vi "DAQNavi Read (Counter 1D Pulse Width 1Chan NSamp).vi"(8 "error in (no error)":errorcluster, 9 "number of samples per channel to read":u32=10, 10 "timeout":dbl=10.0, 11 "task in":i32) -> (0 "error out":errorcluster, 2 "data":cluster{"high period":dbl, "low period":dbl}[](array[cluster]), 3 "task out":i32)   [LabVIEW 2020]
uses:
  DAQNavi_LV.dll
panel:
  in  "pulse width 2":cluster{"high period":dbl, "low period":dbl}
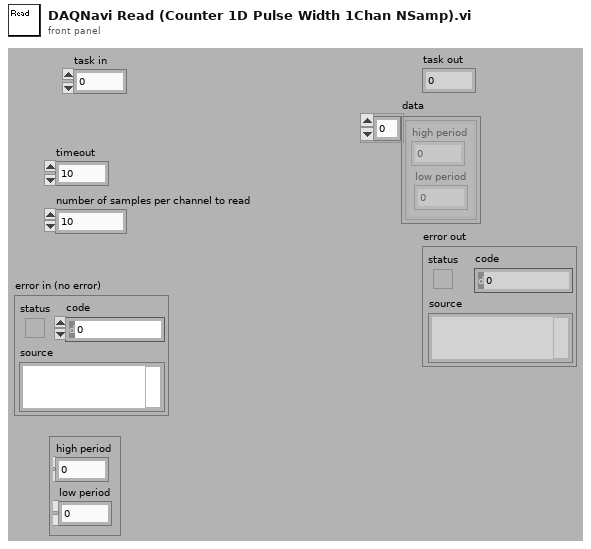
[diagram p1: front panel]
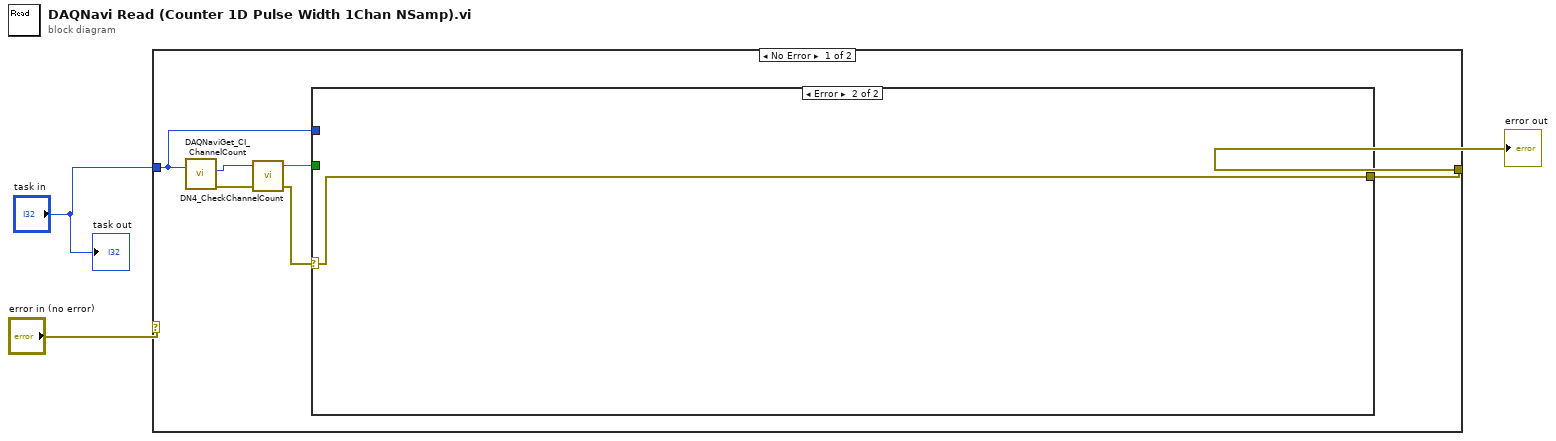
[diagram p0: block diagram]
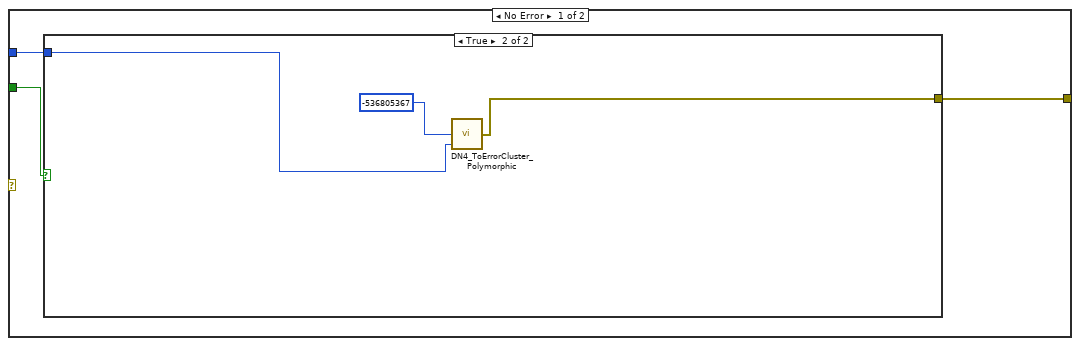
[diagram p2: hidden frame]
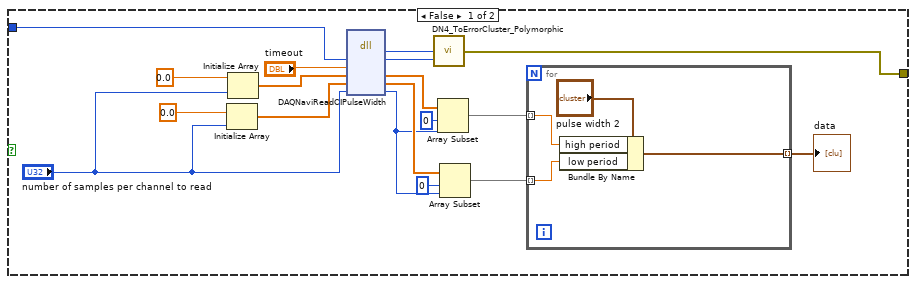
[diagram p3: hidden frame]
diagram:
  n1 = case shown="No Error" "error in (no error)" {
    selector: "error in (no error)" -> [_ w39]
    tunnel: [w9 w39] -> w2
    tunnel: "task in" -> [w4 _]
    frame No Error {
      n2 = call "DAQNaviGet_CI_ChannelCount.vi"("task in"=w4) -> ("error out"=w7:errorcluster, "channel count"=w8:i32)  [unwired: 1 in, 8 out]
      n3 = call "DN4_CheckChannelCount.vi"("error out"=w7, "channel count"=w8) -> ("error IO"=w6:errorcluster, "greater than 1?"=w5:bool)  [unwired: 2 out]
      n4 = case shown="Error" w6 {
        selector: w6 -> [_ w38]
        tunnel: [w12 w38] -> w9
        tunnel: w5 -> [w11 _]
        tunnel: w4 -> [w10 _]
        frame No Error {
          n5 = case shown="True" w11 {
            tunnel: [w14 w35] -> w12
            tunnel: w10 -> [w13 w36]
            frame False {
              n6 = Initialize Array(0.0 ("element"), "number of samples per channel to read") -> (w20:dbl[])
              n7 = Initialize Array(0.0 ("element"), "number of samples per channel to read") -> (w21:dbl[])
              n8 = dll-call lib="DAQNavi_LV.dll" fn="DAQNaviReadCIPulseWidth"("taskID"=w13, "timeout"="timeout", "hiPeriod"=w21, "loPeriod"=w20, "samples"="number of samples per channel to read") -> ("return type"=w30:i32, "taskID"=w15:i32, "hiPeriod"=w25:dbl[], "loPeriod"=w27:dbl[], "samples"=w16:u32)  [unwired: 4 in, 2 out]
              n9 = call "DN4_ToErrorCluster_Polymorphic.vi"("task id"=w15, "error code"=w30) -> ("error out"=w14:errorcluster)  [unwired: 3 out]
              n10 = Array Subset(array=w25, index=0, length=w16) -> (w19:dbl[])
              n11 = Array Subset(array=w27, index=0, length=w16) -> (w18:dbl[])
              n12 = for {
                tunnel: w19 -> [w34] mode=indexing
                tunnel: w18 -> [w33] mode=indexing
                tunnel: [w32] -> w17 mode=indexing
                n13 = Bundle By Name(cluster="pulse width 2", "high period"=w34, "low period"=w33) -> (w32:cluster{"high period":dbl, "low period":dbl})
              }
              "data" <- w17
            }
            frame True {
              n14 = call "DN4_ToErrorCluster_Polymorphic.vi"("task id"=w36, "error code"=-536805367 ("error code (0)")) -> ("error out"=w35:errorcluster)  [unwired: 3 out]
            }
          }
        }
        frame Error {
        }
      }
    }
    frame Error {
    }
  }
  "error out" <- w2
  "task out" <- "task in"
